vi "uActor_RESERVED.vi"(6 "Original uMsg":refnum<class "uMsg.lvclass">, 8 "error in (no error)":errorcluster, 9 "Data":refnum<class "uData.lvclass">, 10 "Command":string, 11 "uActor in":refnum<class "uActor.lvclass">) -> (0 "error out":errorcluster, 1 "reply":refnum<class "uData.lvclass">, 3 "uActor out":refnum<class "uActor.lvclass">)   [LabVIEW 2021, in "uFramework.lvlib" / "uActor.lvclass"]
doc: "This is a reserved space for architectural-critical messages. It is used where children cannot use the normal EXEC method because critical funtions will breakdown if the grandchildren override the EXEC method.\n\nThe parent method returns an error if it receives an unknown incoming command."
uses:
  uActor.lvclass
  Bin/uData.lvlibp/uData.lvclass
  uMsg/uMsg.lvclass
  <vilib>/Utility/error.llb/Error Cluster From Error Code.vi
  <vilib>/ErrorRing/Error Ring.xnode
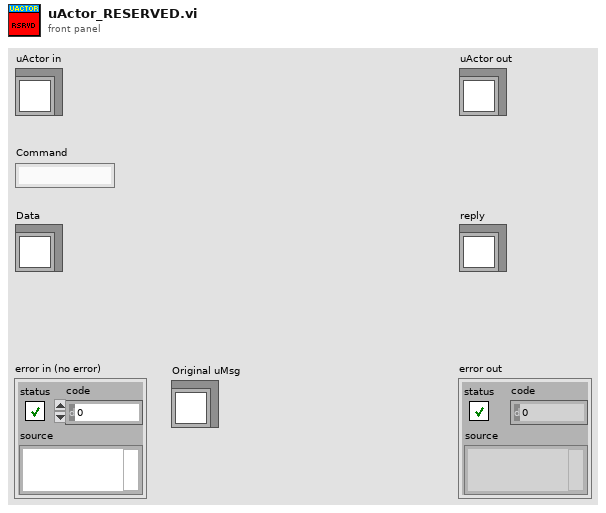
[diagram p1: front panel]
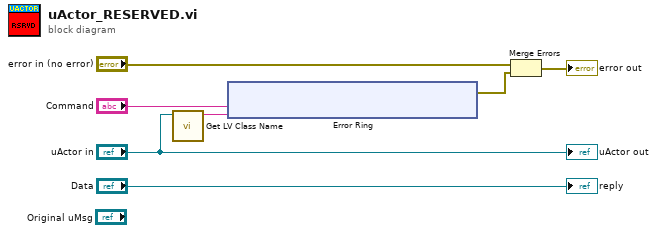
[diagram p0: block diagram]
diagram:
  n1 = call <vilib>:"Get LV Class Name.vi"("object"="uActor in") -> ("class name"=w2:string)  [unwired: 9 in, 1 out]
  n2 = xnode "Error Ring"("parameter 0"="Command", "parameter 1"=w2) -> ("error out"=w5:errorcluster)
  n3 = Merge Errors("error in (no error)", w5) -> (→"error out":errorcluster)
  "uActor out" <- "uActor in"
  "reply" <- "Data"
